vi "Lightning Teleop.vi"(11 "rt fifo":refnum<k33>) -> ()   [LabVIEW 2013]
uses:
  dashboard/TeleopCmd.ctl
  <vilib>/Rock Robotics/WPI/Joystick/WPI_JoystickGetSetRefNum.vi
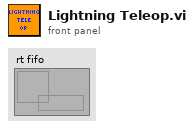
[diagram p1: front panel]
types:
  T1 = typedef "TeleopCmd.ctl" = cluster{"Left Joystick":dbl, "Right Joystick":dbl, "Shift":bool}
  T2 = typedef "WPI_JoystickDevRef.ctl" = cluster{"Device":T3}
  T3 = typedef "WPI_JoystickDeviceEnum.ctl" = enum16{"USB 1", "USB 2", "USB 3", "USB 4", "Kinect 1", "Kinect 2"}
  T4 = typedef "WPI_JoystickButtonState.ctl" = cluster{"Button 1":bool, "Button 2":bool, "Button 3":bool, "Button 4":bool, "Button 5":bool, "Button 6":bool, "Button 7":bool, "Button 8":bool, "Button 9":bool, "Button 10":bool, "Button 11":bool, "Button 12":bool}
  T5 = cluster{"axis 1 (x)":dbl, "axis 2 (y)":dbl, "axis 3 (throttle)":dbl, "axis 4":dbl, "axis 5":dbl, "axis 6":dbl}
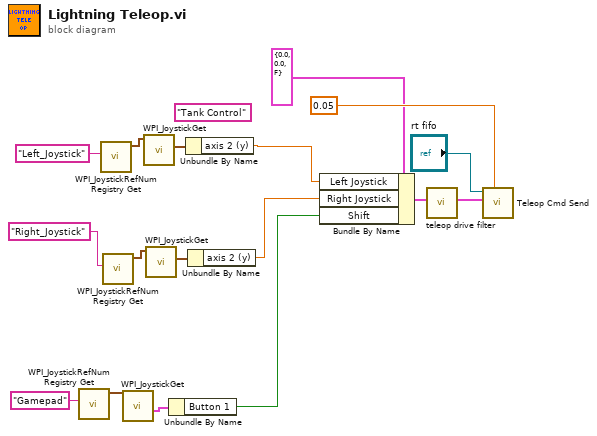
[diagram p0: block diagram]
diagram:
  (unwired) "Tank Control" ("Notifier Name")
  n1 = call <vilib>:"WPI_JoystickRefNum Registry Get.vi"("refnum name"="Gamepad") -> ("JoystickDevRef"=w9:T2)  [unwired: 9 in, 1 out]
  n2 = call <vilib>:"WPI_JoystickRefNum Registry Get.vi"("refnum name"="Left_Joystick") -> ("JoystickDevRef"=w13:T2)  [unwired: 9 in, 1 out]
  n3 = call <vilib>:"WPI_JoystickRefNum Registry Get.vi"("refnum name"="Right_Joystick") -> ("JoystickDevRef"=w16:T2)  [unwired: 9 in, 1 out]
  n4 = call <vilib>:"WPI_JoystickGet.vi"("JoystickDevRef"=w9) -> ("Buttons"=w10:T4)  [unwired: 4 in, 2 out]
  n5 = call <vilib>:"WPI_JoystickGet.vi"("JoystickDevRef"=w13) -> ("Axes"=w14:T5)  [unwired: 4 in, 2 out]
  n6 = call <vilib>:"WPI_JoystickGet.vi"("JoystickDevRef"=w16) -> ("Axes"=w17:T5)  [unwired: 4 in, 2 out]
  n7 = Unbundle By Name(w10) -> ("Button 1"=w4:bool)
  n8 = Unbundle By Name(w14) -> ("axis 2 (y)"=w6:dbl)
  n9 = Unbundle By Name(w17) -> ("axis 2 (y)"=w5:dbl)
  n10 = Bundle By Name(cluster=T1 {"Left Joystick"=0.0, "Right Joystick"=0.0, "Shift"=FALSE} ("Cluster"), "Left Joystick"=w6, "Right Joystick"=w5, "Shift"=w4) -> (w2:T1)
  n11 = call "teleop drive filter.vi"("input data"=w2) -> ("output data"=w1:T1)  [unwired: 10 in]
  n12 = call "Teleop Cmd Send.vi"("rt fifo"="rt fifo", "Cluster"=w1, "Epsilon"=0.05) -> ()  [unwired: 7 in, 1 out]
